vi "SpotFinderIngoHeucke.vi"(1 "auto":bool, 4 "Int duplex?":refnum<vi>, 5 "notes":refnum<vi>, 6 "router 3":refnum<vi>, 7 "plane 2":refnum<vi>, 8 "Image Path":refnum<vi>, 9 "16bit?":refnum<vi>, 10 "TACwinLoaded?":refnum<vi>) -> ()   [LabVIEW 2009]
panel:
  out "already x spots":i16
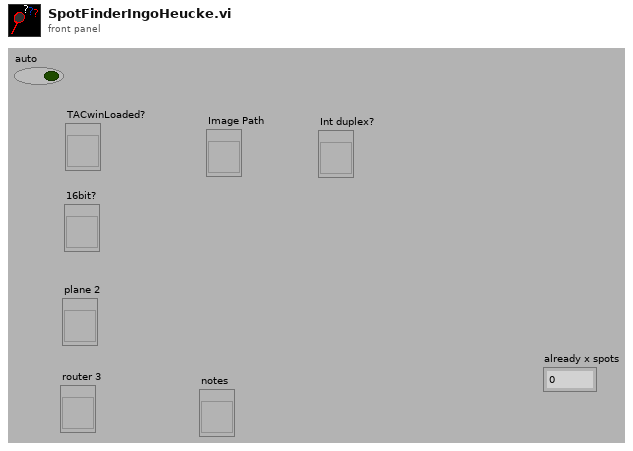
[diagram p1: front panel]
types:
  T1 = enum16{"Ini", "Dump", "Colorpal", "Input", "Get"}
  T2 = enum16{"Display", "change", "get", "save", "create text", "load", "Get Refnum"}
  T3 = enum16{"Ini", "Get", "Set", "Refresh", "dump", "move", "name"}
  T4 = typedef "spotproperties.ctl" = cluster{"draw?":bool, "plane":u32, "Coordinates":i32[], "TACWindow":cluster{"TACWindow1":i32, "TACWindow2":i32}, "Lifetime[ns]":ext[], "tauerror":dbl[], "F2-Value overall":dbl, "overall intensity":u32[], "F2-Value TAC":dbl, "TAC intensity":u32[], "Decay":u32[][]}
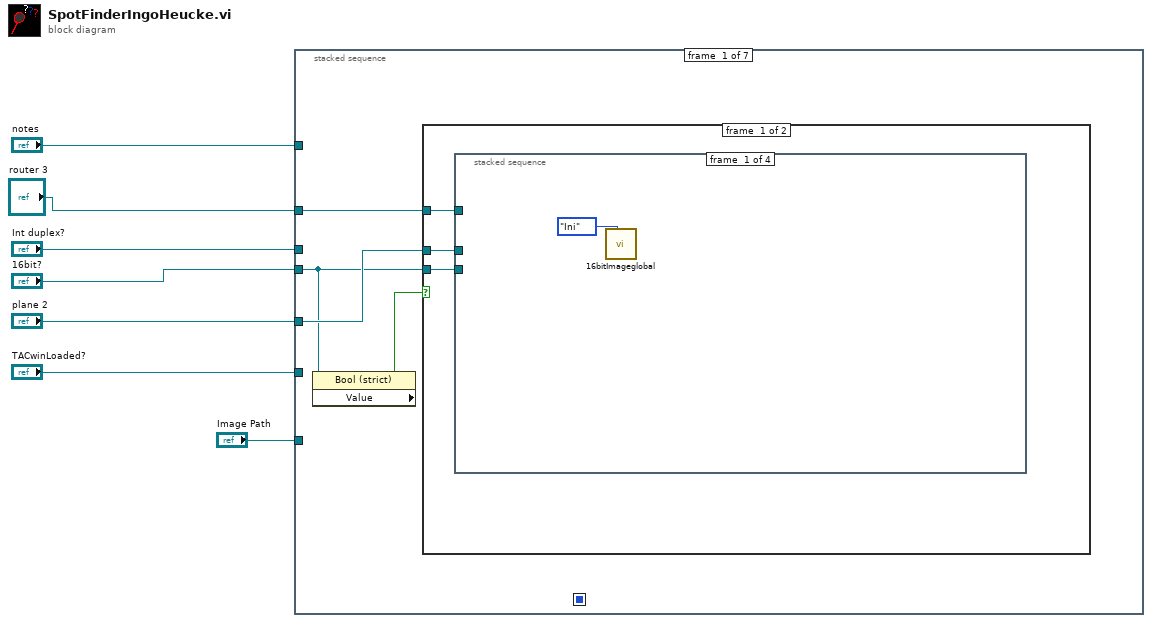
[diagram p0: block diagram]
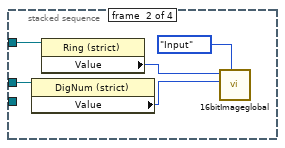
[diagram p2: hidden frame]
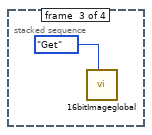
[diagram p3: hidden frame]
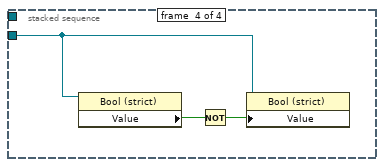
[diagram p4: hidden frame]
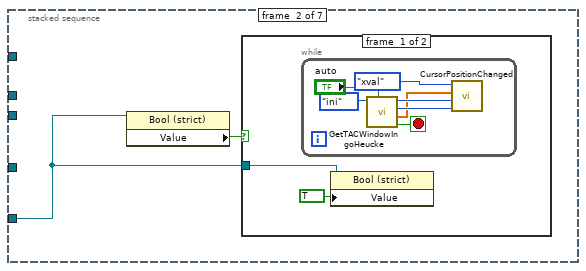
[diagram p6: hidden frame]
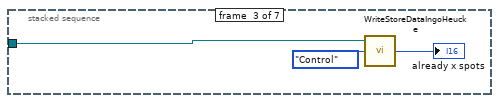
[diagram p8: hidden frame]
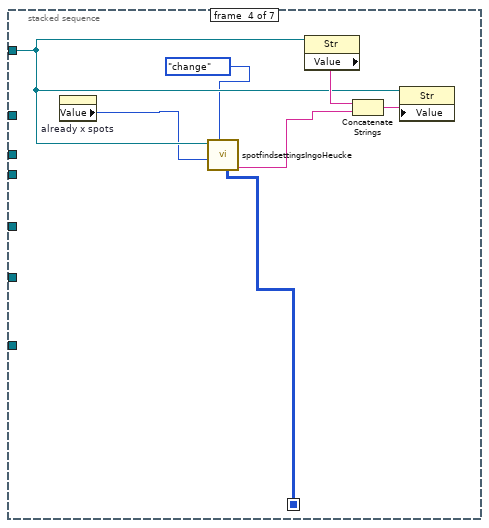
[diagram p9: hidden frame]
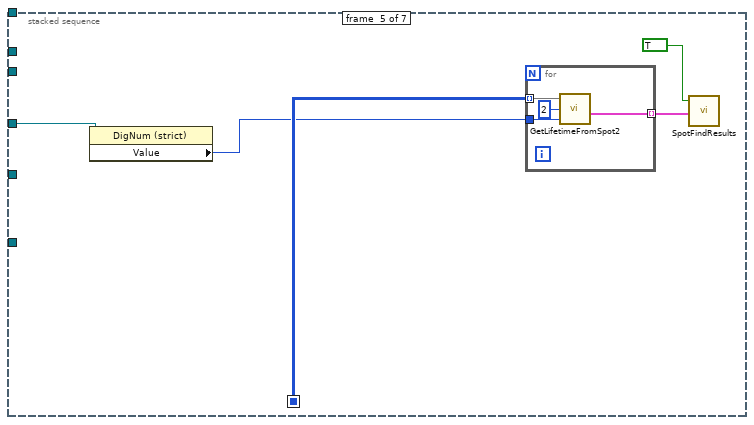
[diagram p10: hidden frame]
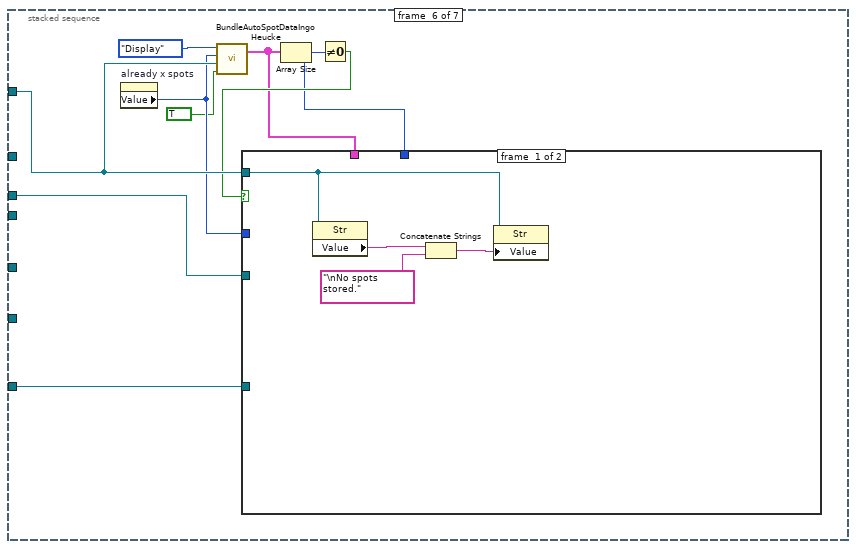
[diagram p11: hidden frame]
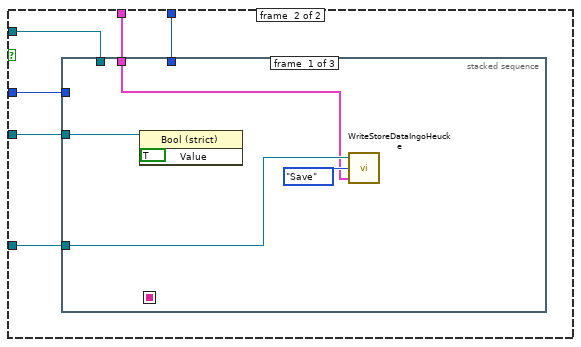
[diagram p12: hidden frame]
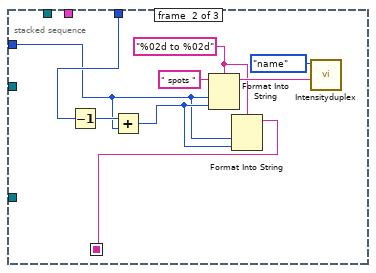
[diagram p13: hidden frame]
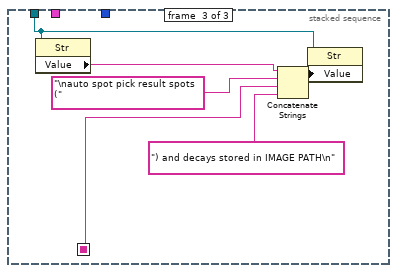
[diagram p14: hidden frame]
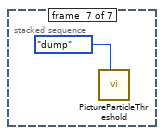
[diagram p15: hidden frame]
diagram:
  n1 = stacked-sequence {
    seq-local: [_ _ _ w39 _ _ _] -> [_ _ _ _ w50 _ _]
    tunnel: "TACwinLoaded?" -> [_ w25 _ _ _ _ _]
    tunnel: "router 3" -> [w10 _ _ _ _ _ _]
    tunnel: "plane 2" -> [w9 _ _ _ w49 _ _]
    tunnel: "16bit?" -> [w8 _ _ _ _ _ _]
    tunnel: "Int duplex?" -> [_ _ _ _ _ w63 _]
    tunnel: "notes" -> [_ _ _ w43 _ w61 _]
    tunnel: "Image Path" -> [_ _ w37 _ _ w62 _]
    frame #0 {
      n2 = property on="Property Node" class="Bool (strict)"(reference=w8) -> ("Value"=w11:bool)  [unwired: 1 in, 2 out]
      n3 = case shown="False" w11 {
        tunnel: w10 -> [w14 _]
        tunnel: w9 -> [w13 _]
        tunnel: w8 -> [w12 _]
        frame #0 {
          n4 = stacked-sequence {
            tunnel: w14 -> [_ w17 _ _]
            tunnel: w13 -> [_ w16 _ _]
            tunnel: w12 -> [_ _ _ w22]
            frame #0 {
              n5 = call "16bitImageglobal.vi"("Enum"=T1."Ini") -> ()  [unwired: 4 in, 4 out]
            }
            frame #1 {
              n6 = property on="Property Node" class="DigNum (strict)"(reference=w16) -> ("Value"=w19:u32)  [unwired: 1 in, 2 out]
              n7 = property on="Property Node" class="Ring (strict)"(reference=w17) -> ("Value"=w20:u8)  [unwired: 1 in, 2 out]
              n8 = call "16bitImageglobal.vi"("Enum"=T1."Input", "plane"=w19, "router"=w20) -> ()  [unwired: 2 in, 4 out]
            }
            frame #2 {
              n9 = call "16bitImageglobal.vi"("Enum"=T1."Get") -> ()  [unwired: 4 in, 4 out]
            }
            frame #3 {
              n10 = property on="Property Node" class="Bool (strict)"(reference=w22) -> ("Value"=w24:bool)  [unwired: 1 in, 2 out]
              n11 = Not(x=w24) -> (.not. x?=w23:bool)
              n12 = property on="Property Node" class="Bool (strict)"(reference=w22, "Value"=w23) -> ()  [unwired: 1 in, 2 out]
            }
          }
        }
        frame #1 {
        }
      }
    }
    frame #1 {
      n13 = property on="Property Node" class="Bool (strict)"(reference=w25) -> ("Value"=w26:bool)  [unwired: 1 in, 2 out]
      n14 = case shown="False" w26 {
        tunnel: w25 -> [w27 _]
        frame #0 {
          n15 = while {
            stop <- w34 stop-if-true
            n16 = call "GetTACWindowIngoHeucke.vi"("Enum"=enum16{"ini", "get", "quick"}."ini", "auto"="auto") -> ("Cursor.Cursor Position:Cursor X"=w33:u16, "Cursor.Cursor Position:Cursor X 2"=w32:u16, "x-values"=w30:dbl[], "ready?"=w34:bool)  [unwired: 5 out]
            n17 = call "CursorPositionChanged.vi"("CursorPos x1"=w32, "CursorPos x0"=w33, "x-values"=w30, "action"=enum16{"Check", "Get", "xval"}."xval" ("Enum")) -> ()  [unwired: 4 out]
          }
          n18 = property on="Property Node" class="Bool (strict)"(reference=w27, "Value"=TRUE) -> ()  [unwired: 1 in, 2 out]
        }
        frame #1 {
        }
      }
    }
    frame #2 {
      n19 = call "WriteStoreDataIngoHeucke.vi"("Enum"=enum16{"Save", "Control"}."Control", "Image Path"=w37) -> ("already x spots"=→"already x spots":i16)  [unwired: 1 in]
    }
    frame #3 {
      n20 = property on="already x spots" class="Digital (strict)"() -> ("Value"=w42:i16)  [unwired: 2 in, 2 out]
      n21 = call "spotfindsettingsIngoHeucke.vi"("Enum"=T2."change", "already x spots found"=w42, "notes 2"=w43) -> ("settings"=w40:string, "coordinates"=w39:i32[][])  [unwired: 6 in, 1 out]
      n22 = property on="Property Node" class="Str"(reference=w43) -> ("Value"=w45:string)  [unwired: 1 in, 2 out]
      n23 = Concatenate Strings(w45, w40) -> (w44:string)
      n24 = property on="Property Node" class="Str"(reference=w43, "Value"=w44) -> ()  [unwired: 1 in, 2 out]
    }
    frame #4 {
      n25 = property class="DigNum (strict)"(reference=w49) -> ("Value"=w48:u32)  [unwired: 1 in, 2 out]
      n26 = for {
        tunnel: w50 -> [w54] mode=indexing
        tunnel: [w53] -> w46 mode=indexing
        tunnel: w48 -> [w52]
        n27 = call "GetLifetimeFromSpot2.vi"("plane"=w52, "F2-channel"=u8 2, "Coordinates"=w54) -> ("SpotProperties"=w53:T4)  [unwired: 5 in]
      }
      n28 = call "SpotFindResults.vi"("Spots in"=w46, "set?"=TRUE) -> ()  [unwired: 3 in, 1 out]
    }
    frame #5 {
      n29 = property on="already x spots" class="Digital (strict)"() -> ("Value"=w56:i16)  [unwired: 2 in, 2 out]
      n30 = call "BundleAutoSpotDataIngoHeucke.vi"("auto"=TRUE, "notes 2"=w61, "already x spots"=w56, "Enum"=enum16{"1st sort", "Display", "Get"}."Display") -> ("Spots out"=w58:T4[])  [unwired: 1 in]
      n31 = Array Size(array=w58) -> (size(s)=w57:i32)
      n32 = Not Equal To 0?(x=w57) -> (x != 0?=w59:bool)
      n33 = case shown="True" w59 {
        tunnel: w58 -> [_ w73]
        tunnel: w57 -> [_ w72]
        tunnel: w63 -> [_ w71]
        tunnel: w61 -> [w64 w70]
        tunnel: w56 -> [_ w69]
        tunnel: w62 -> [_ w68]
        frame #0 {
          n34 = property on="Property Node" class="Str"(reference=w64) -> ("Value"=w67:string)  [unwired: 1 in, 2 out]
          n35 = Concatenate Strings(w67, "\nNo spots stored." ("string")) -> (w66:string)
          n36 = property on="Property Node" class="Str"(reference=w64, "Value"=w66) -> ()  [unwired: 1 in, 2 out]
        }
        frame #1 {
          n37 = stacked-sequence {
            seq-local: [_ w82 _] -> [_ _ w89]
            tunnel: w73 -> [w74 _ _]
            tunnel: w72 -> [_ w80 _]
            tunnel: w71 -> [w76 _ _]
            tunnel: w70 -> [_ _ w88]
            tunnel: w69 -> [_ w79 _]
            tunnel: w68 -> [w75 _ _]
            frame #0 {
              n38 = property on="Property Node" class="Bool (strict)"(reference=w76, "Value"=TRUE ("Boolean 2")) -> ()  [unwired: 1 in, 2 out]
              n39 = call "WriteStoreDataIngoHeucke.vi"("Spots"=w74, "Enum"=enum16{"Save", "Control"}."Save", "Image Path"=w75) -> ()  [unwired: 1 out]
            }
            frame #1 {
              w84 = "%02d to %02d" ("format string")
              n40 = Decrement(x=w80) -> (x-1=w83:i32)
              n41 = Add(x=w83, y=w79) -> (x+y=w81:i32)
              n42 = Format Into String(format string=w84, initial string=" spots ", w79, w81) -> (resulting string=w85:string)  [unwired: 1 in, 1 out]
              n43 = Format Into String(format string=w84, w79, w81) -> (resulting string=w82:string)  [unwired: 2 in, 1 out]
              n44 = call "Intensityduplex.vi"("Enum"=T3."name", "add string"=w85) -> ()  [unwired: 3 in, 2 out]
            }
            frame #2 {
              n45 = property on="Property Node" class="Str"(reference=w88) -> ("Value"=w92:string)  [unwired: 1 in, 2 out]
              n46 = Concatenate Strings(w92, "\nauto spot pick result spots (" ("string"), w89, ") and decays stored in IMAGE PATH\n" ("string")) -> (w91:string)
              n47 = property on="Property Node" class="Str"(reference=w88, "Value"=w91) -> ()  [unwired: 1 in, 2 out]
            }
          }
        }
      }
    }
    frame #6 {
      n48 = call "PictureParticleThreshold.vi"("Enum"=enum16{"new", "input", "draw", "dump"}."dump") -> ()  [unwired: 7 in, 2 out]
    }
  }
